vi "Create.vi"(8 "error in":errorcluster, 10 "Node":refnum<k20>, 11 "Node in":refnum<class "Node.lvclass">) -> (0 "error out":errorcluster, 3 "Node out":refnum<class "Node.lvclass">)   [LabVIEW 2014, in "Node.lvclass"]
uses:
  Node.lvclass
  Node.lvclass/Node.ctl
  <resource>/objmgr/DOMUserDefRef.rc
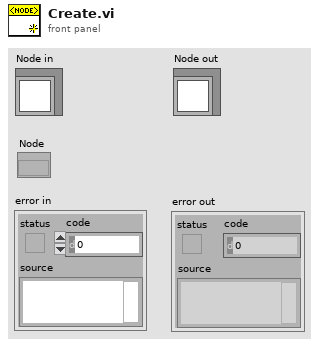
[diagram p1: front panel]
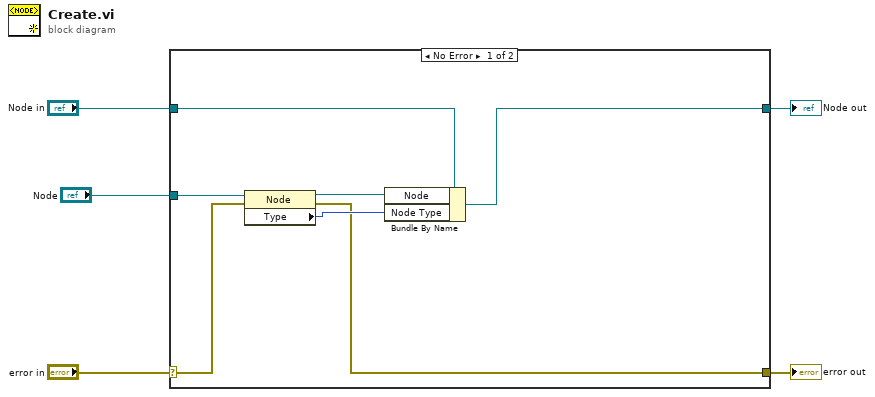
[diagram p0: block diagram]
diagram:
  n1 = case shown="No Error" "error in" {
    selector: "error in" -> [w7 w14]
    tunnel: [w6 w14] -> w4
    tunnel: [w11 w13] -> w2
    tunnel: "Node in" -> [w12 w13]
    tunnel: "Node" -> [w10 _]
    frame No Error {
      n2 = property class="Node"(reference=w10, error in=w7) -> (reference out=w9:refnum<k20>, error out=w6:errorcluster, "Type"=w8:i32)
      n3 = Bundle By Name(cluster=w12, "Node"=w9, "Node Type"=w8) -> (w11:refnum<class "Node.lvclass">)
    }
    frame Error {
    }
  }
  "error out" <- w4
  "Node out" <- w2
